vi "SubVI_Prescan Run.vi"(8 "error in (no error)":errorcluster, 11 "VISA in":refnum<visa-resource-name>) -> (0 "error out":errorcluster, 1 "Raw data 1D array":dbl[](array[numeric]), 2 "Frequency VS Amplitude (2D array)":dbl[][](array[numeric]), 3 "VISA out":refnum<visa-resource-name>)   [LabVIEW 2016]
doc: "Fetch binary trace from Spec An, output 2D trace array with frequency VS amplitude (X vs Y) information"
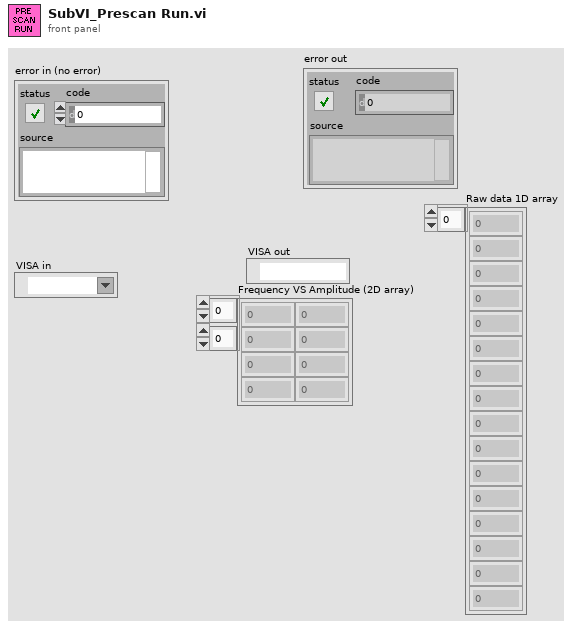
[diagram p1: front panel]
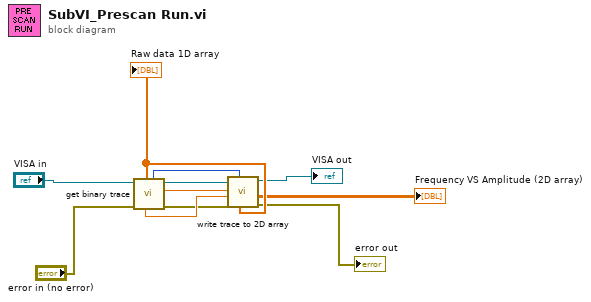
[diagram p0: block diagram]
diagram:
  n1 = call "get binary trace.vi"("error in (no error)"="error in (no error)", "VISA resource in"="VISA in") -> ("error out"=w5:errorcluster, "Start frequency (Hz)"=w11:dbl, "VISA resource out"=w7:refnum<visa-resource-name>, "Number of points"=w8:i32, "Linear frequecny increment (Hz)"=w9:dbl, "Trace Array (1D)"=w6:dbl[])  [unwired: 2 in, 1 out]
  "Raw data 1D array" <- w6
  n2 = call "write trace to 2D array.vi"("Input array"=w6, "Number of points"=w8, "error in (no error)"=w5, "Linear Increment (MHz)"=w9, "Start F (MHz)"=w11, "Visa in"=w7) -> ("error out"=→"error out":errorcluster, "Frequency VS Amplitude (2D array)"=→"Frequency VS Amplitude (2D array)":dbl[][], "VISA resource name"=→"VISA out":refnum<visa-resource-name>)  [unwired: 1 in, 2 out]
